vi "test_TCP_Open connection using Clear Error node.vi"(8 "error in (no error)":errorcluster, 11 "TestCase in":refnum<class "Ethernet Protocol Tests.lvclass">) -> (0 "error out":errorcluster, 3 "TestCase out":refnum<class "Ethernet Protocol Tests.lvclass">)   [LabVIEW 2019, in "Ethernet Protocol Tests.lvclass"]
uses:
  Ethernet Protocol Tests.lvclass
  TCP/TCP.lvclass
  TCP/TCP.lvclass/TCP.ctl
  <vilib>/addons/_JKI Toolkits/VI Tester/TestCase.llb/TestCase.lvclass
  C:/Program Files (x86)/National Instruments/LabVIEW 2019/vi.lib/addons/_JKI Toolkits/VI Tester/TestCase.llb/TestCase.lvclass
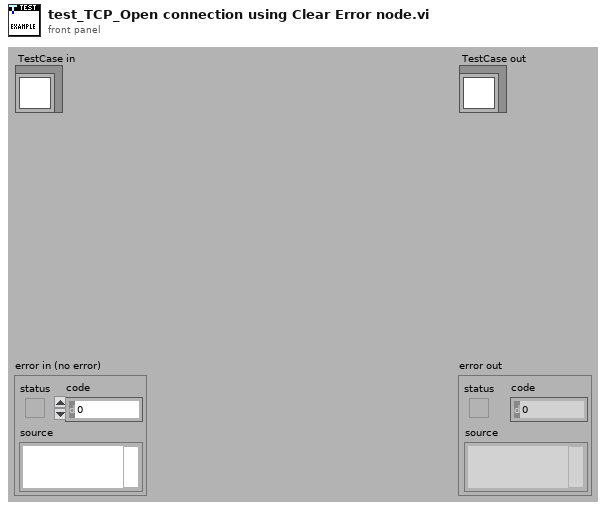
[diagram p1: front panel]
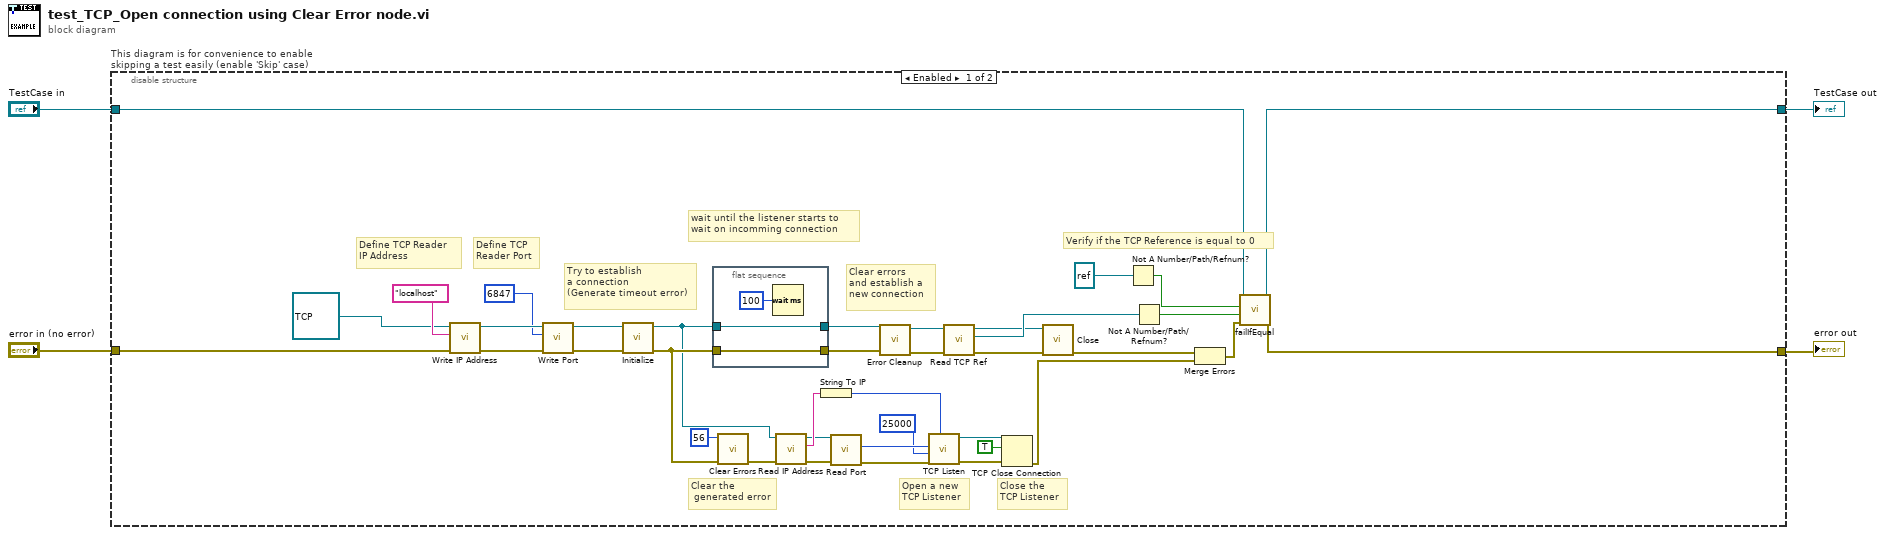
[diagram p0: block diagram]
diagram:
  n1 = disable-structure "This diagram is for convenience to enable skipping a test easily (enable 'Skip' case)" shown="Enabled" {
    disable-tunnel: "TestCase in" -> [w42 w49]
    disable-tunnel: [w15 w47] -> w1
    disable-tunnel: [w14 w48] -> w3
    disable-tunnel: "error in (no error)" -> [w36 w46]
    frame Enabled {
      # "Verify if the TCP Reference is equal to 0"
      # "Clear the\n generated error"
      # "Close the \nTCP Listener"
      # "Open a new \nTCP Listener"
      # "Clear errors \nand establish a \nnew connection"
      # "Try to establish \na connection\n(Generate timeout error)"
      # "wait until the listener starts to\nwait on incomming connection"
      # "Define TCP \nReader Port"
      # "Define TCP Reader \nIP Address"
      n2 = call "Write IP Address.vi"("error in (no error)"=w36, "IP Address"="localhost", "Ethernet in"=refnum<class "TCP.lvclass"> refnum ("Protocols.lvlib:TCP.lvclass")) -> ("error out"=w39:errorcluster, "Ethernet out"=w40:refnum<class "TCP.lvclass">)  [unwired: 7 in]
      n3 = call "Write Port.vi"("error in (no error)"=w39, "Port"=u16 6847, "Ethernet in"=w40) -> ("error out"=w35:errorcluster, "Ethernet out"=w34:refnum<class "TCP.lvclass">)  [unwired: 7 in]
      n4 = call-dynamic "Initialize.vi"("error in (no error)"=w35, "Ethernet in"=w34) -> ("error out"=w23:errorcluster, "Ethernet out"=w22:refnum<class "TCP.lvclass">)  [unwired: 8 in]
      n5 = flat-sequence {
        tunnel: w23 -> [w45]
        tunnel: w22 -> [w44]
        tunnel: [w45] -> w26
        tunnel: [w44] -> w25
        frame #0 {
          n6 = Wait (ms)(milliseconds to wait=u32 100) -> ()  [unwired: 1 out]
        }
      }
      n7 = call <vilib>:"Clear Errors.vi"("error in (no error)"=w23, "specific error code to clear (0: all)"=56) -> ("error out"=w24:errorcluster)  [unwired: 4 in, 1 out]
      n8 = call "Read IP Address.vi"("error in (no error)"=w24, "Ethernet in"=w22) -> ("error out"=w31:errorcluster, "IP Address"=w33:string, "Ethernet out"=w30:refnum<class "TCP.lvclass">)  [unwired: 7 in]
      n9 = String To IP(1:w33) -> (0:w32:u32)
      n10 = call "Read Port.vi"("error in (no error)"=w31, "Ethernet in"=w30) -> ("error out"=w29:errorcluster, "Port"=w28:u16)  [unwired: 7 in, 1 out]
      n11 = call-dynamic "Error Cleanup.vi"("error in (no error)"=w26, "Ethernet in"=w25) -> ("error out"=w13:errorcluster, "Ethernet out"=w12:refnum<class "TCP.lvclass">)  [unwired: 8 in]
      n12 = call <vilib>:"TCP Listen.vi"("net address"=w32, "error in (no error)"=w29, "timeout ms (wait forever: -1)"=25000, "port"=w28) -> ("error out"=w20:errorcluster, "connection ID"=w19:refnum<k5>)  [unwired: 3 in, 3 out]
      n13 = call "Read TCP Ref.vi"("error in (no error)"=w13, "Ethernet in"=w12) -> ("error out"=w7:errorcluster, "TCP Ref"=w11:refnum<k5>, "Ethernet out"=w5:refnum<class "TCP.lvclass">)  [unwired: 7 in]
      n14 = TCP Close Connection(connection ID=w19, abort (F)=TRUE, error in (no error)=w20) -> (error out=w17:errorcluster)  [unwired: 1 out]
      n15 = call-dynamic "Close.vi"("error in (no error)"=w7, "Ethernet in"=w5) -> ("error out"=w6:errorcluster)  [unwired: 8 in, 1 out]
      n16 = Not A Number/Path/Refnum?(number/path/refnum=refnum<k5> refnum ("TCP Ref")) -> (NaN/Path/Refnum?=w8:bool)
      n17 = Not A Number/Path/Refnum?(number/path/refnum=w11) -> (NaN/Path/Refnum?=w10:bool)
      n18 = Merge Errors(w6, w17) -> (w16:errorcluster)
      n19 = call-dynamic "failIfEqual.vi"("error in (no error)"=w16, "y"=w10, "x"=w8, "TestCase in"=w42) -> ("error out"=w14:errorcluster, "TestCase out"=w15:refnum<class "Ethernet Protocol Tests.lvclass">)  [unwired: 6 in]
    }
    frame Disabled {
      # "skip test result while test is under development"
      n20 = call <vilib>:"skip.vi"("error in (no error)"=w46, "TestCase in"=w49) -> ("error out"=w48:errorcluster, "TestCase out"=w47:refnum<class "Ethernet Protocol Tests.lvclass">)  [unwired: 8 in]
    }
  }
  "error out" <- w3
  "TestCase out" <- w1
